vi "Arcade Drive.vi"(10 "Drive":dbl, 11 "Rotate":dbl) -> (0 "Left Motor":i8, 1 "Right Motor":i8)   [LabVIEW 2016]
uses:
  <vilib>/NXT/Dual Mode Library/prims/inRangeAndCoerce/inRangeAndCoerce_float.vi
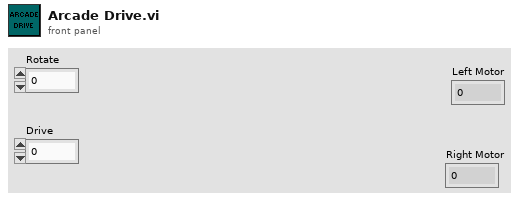
[diagram p1: front panel]
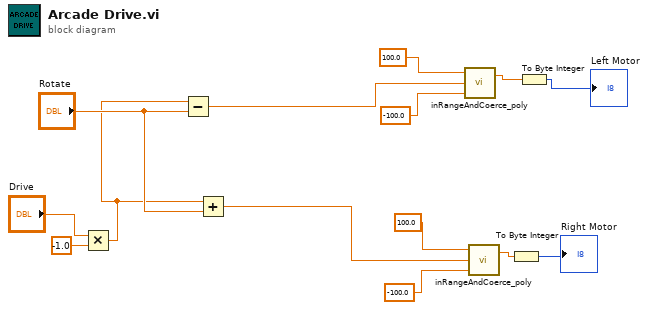
[diagram p0: block diagram]
diagram:
  n1 = Multiply(x="Drive", y=-1.0) -> (x*y=w2:dbl)
  n2 = Subtract(x=w2, y="Rotate") -> (x-y=w5:dbl)
  n3 = Add(x=w2, y="Rotate") -> (x+y=w4:dbl)
  n4 = call-poly <vilib>:"inRangeAndCoerce_poly.vi"("lower limit"=sgl -100.0, "x"=w5, "upper limit"=sgl 100.0) -> ("coerced(x)"=w8:sgl)  [unwired: 1 out]
  n5 = call-poly <vilib>:"inRangeAndCoerce_poly.vi"("lower limit"=sgl -100.0, "x"=w4, "upper limit"=sgl 100.0) -> ("coerced(x)"=w9:sgl)  [unwired: 1 out]
  n6 = To Byte Integer(number=w9) -> (8bit integer=→"Right Motor":i8)
  n7 = To Byte Integer(number=w8) -> (8bit integer=→"Left Motor":i8)
